vi "Field Relative Swerve.vi"(8 "Field Relative Active":bool, 10 "PigeonIMUDevRef":T1={"DeviceStatus"={"status"=FALSE, "code"=0, "source"=""}, "Device Number"=0, "Type"=352321536, "Device ID"=0, "Handle"=0, "UsageFrame"=0, "Library Path"=path ""} {"Type" items=["CAN"=352321536, "TalonSRX"=33554432]}, 11 "Axes Magnitudes":cluster{"X":dbl, "Y":dbl, "Z":dbl}) -> (3 "Axes Mag. Changed":cluster{"X":dbl, "Y":dbl, "Z":dbl})   [LabVIEW 2017, in "Huskie Swerve.lvlib"]
uses:
  Huskie Swerve.lvlib
  <vilib>/Rock Robotics/WPI/ThirdParty/Phoenix-LabVIEW/Pigeon IMU/CTRE_PigeonIMU_DeviceRef.ctl
  Public/Documents/Cross The Road Electronics/Phoenix-LabVIEW/Pigeon IMU/CTRE_PigeonIMU_ConnectionType.ctl
  Public/Documents/Cross The Road Electronics/Phoenix-LabVIEW/Pigeon IMU/CTRE_PigeonIMU_GetYPR.vi
  <vilib>/ptbypt/NI_PtbyPt.lvlib
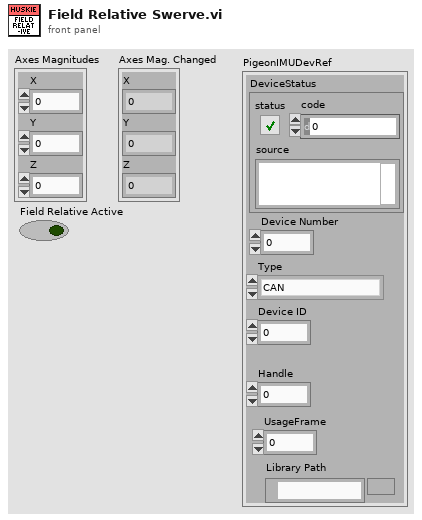
[diagram p1: front panel]
types:
  T1 = typedef "CTRE_PigeonIMU_DeviceRef.ctl" = cluster{"DeviceStatus":errorcluster, "Device Number":u8, "Type":T2, "Device ID":u32, "Handle":u64, "UsageFrame":u32, "Library Path":path}
  T2 = typedef "CTRE_PigeonIMU_ConnectionType.ctl" = u32
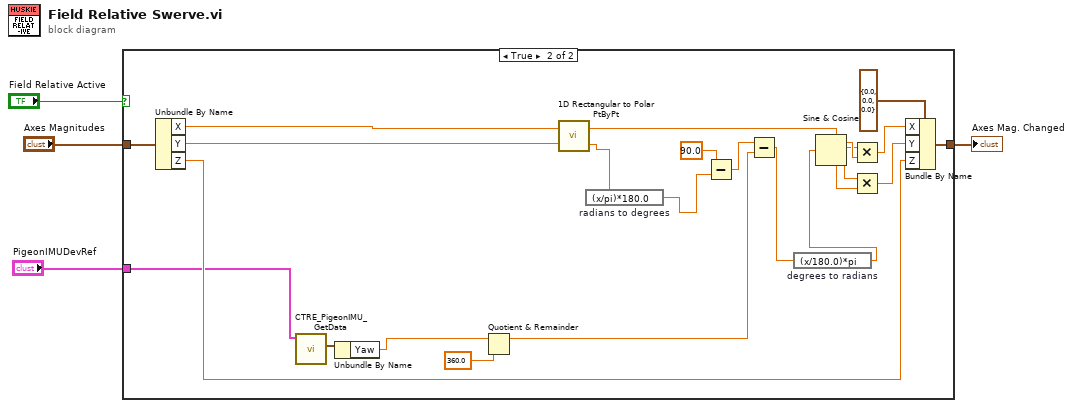
[diagram p0: block diagram]
diagram:
  n1 = case shown="True" "Field Relative Active" {
    tunnel: "Axes Magnitudes" -> [w5 w27]
    tunnel: [w5 w17] -> w3
    tunnel: "PigeonIMUDevRef" -> [_ w6]
    frame False {
    }
    frame True {
      n2 = Unbundle By Name(w27) -> ("X"=w26:dbl, "Y"=w25:dbl, "Z"=w18:dbl)
      n3 = call-poly "CTRE_PigeonIMU_GetData.vi"("PigeonIMUDevRef"=w6) -> ("Yaw Pitch Roll"=w16:cluster{"Yaw":dbl, "Pitch":dbl, "Roll":dbl})  [unwired: 8 in, 2 out]
      n4 = Unbundle By Name(w16) -> ("Yaw"=w14:dbl)
      n5 = Quotient & Remainder(x=w14, y=360.0) -> (x-y*floor(x/y)=w15:dbl)  [unwired: 1 out]
      n6 = call <vilib>:"1D Rectangular to Polar PtByPt.vi"("y"=w25, "x"=w26) -> ("phase"=w12:dbl, "magnitude"=w22:dbl)
      n7 = expression code="(x/pi)*180.0" "radians to degrees"(w12) -> (w11:dbl)
      n8 = Subtract(x=90.0, y=w11) -> (x-y=w9:dbl)
      n9 = Subtract(x=w9, y=w15) -> (x-y=w8:dbl)
      n10 = expression code="(x/180.0)*pi" "degrees to radians"(w8) -> (w7:dbl)
      n11 = Sine & Cosine(0:w7) -> (1:w24:dbl, 2:w23:dbl)
      n12 = Multiply(x=w22, y=w24) -> (x*y=w20:dbl)
      n13 = Multiply(x=w23, y=w22) -> (x*y=w19:dbl)
      n14 = Bundle By Name(cluster=cluster{"X":dbl, "Y":dbl, "Z":dbl} {"X"=0.0, "Y"=0.0, "Z"=0.0} ("Axes Magnitudes 3"), "X"=w20, "Y"=w19, "Z"=w18) -> (w17:cluster{"X":dbl, "Y":dbl, "Z":dbl})
    }
  }
  "Axes Mag. Changed" <- w3
